vi "LCDSetScreenSize.vi"(0 "error in (no error)":errorcluster, 2 "Screen Size":u32(ring)=1 items=["SCREEN_SIZE_NONE"=1, "SCREEN_SIZE_1x8"=2, "SCREEN_SIZE_2x8"=3, "SCREEN_SIZE_1x16"=4, "SCREEN_SIZE_2x16"=5, "SCREEN_SIZE_4x16"=6, "SCREEN_SIZE_2x20"=7, "SCREEN_SIZE_4x20"=8, "SCREEN_SIZE_2x24"=9, "SCREEN_SIZE_1x40"=10, "SCREEN_SIZE_2x40"=11, "SCREEN_SIZE_4x40"=12, "SCREEN_SIZE_64x128"=13], 3 "Device In":u64) -> (7 "error out":errorcluster, 10 "Device Out":u64)   [LabVIEW 2020, in "Phidget LCD.lvlib"]
doc: "${ScreenSize:Header}"
uses:
  <instrlib>/Phidgets/Phidget LCD/Phidget LCD.lvlib
  <instrlib>/Phidgets/Phidget Common/Phidget Common.lvlib
  phidget22.dll
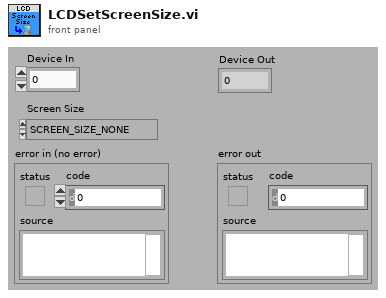
[diagram p1: front panel]
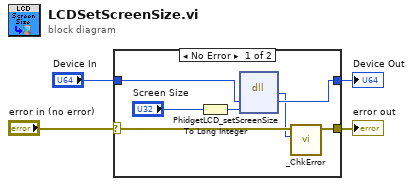
[diagram p0: block diagram]
diagram:
  n1 = case shown="No Error" "error in (no error)" {
    selector: "error in (no error)" -> [w9 w13]
    tunnel: [w8 w13] -> w3
    tunnel: "Device In" -> [w11 w12]
    tunnel: [w10 w12] -> w1
    frame No Error {
      n2 = To Long Integer(number="Screen Size") -> (32bit integer=w5:i32)
      n3 = dll-call lib="phidget22.*" fn="PhidgetLCD_setScreenSize"("phid"=w11, "ScreenSize"=w5) -> ("return type"=w7:i32, "phid"=w10:u64)  [unwired: 4 in, 2 out]
      n4 = call <instrlib>:"_ChkError.vi"("Return Code"=w7, "error in (no error)"=w9) -> ("error out"=w8:errorcluster)  [unwired: 9 in]
    }
    frame Error {
    }
  }
  "error out" <- w3
  "Device Out" <- w1
